vi "相机关闭.vi"(8 "error in (no error)":errorcluster caption="错误输入（无错误）", 11 "数组":T1[](array[typedef])) -> (0 "error out":errorcluster caption="错误输出")   [LabVIEW 2017]
uses:
  <vilib>/userdefined/High Color/IMAQdx.ctl
  <vilib>/vision/driver/NI_Vision_Acquisition_Software.lvlib
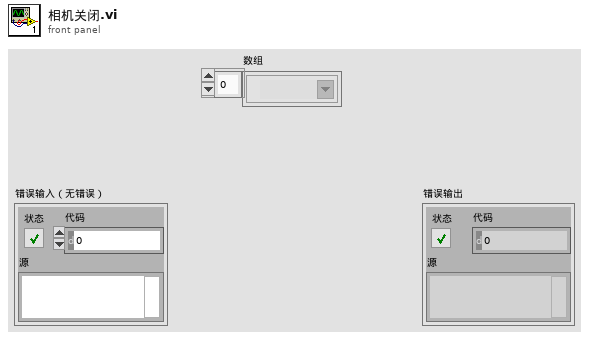
[diagram p1: front panel]
types:
  T1 = typedef "IMAQdx.ctl" = refnum<k21>
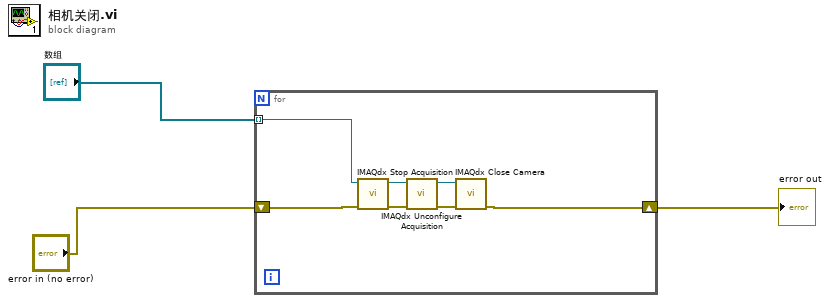
[diagram p0: block diagram]
diagram:
  n1 = for {
    shift-right: [w5] -> w2
    shift-left: "error in (no error)" -> [w6]
    tunnel: "数组" -> [w4] mode=indexing
    n2 = call <vilib>:"IMAQdx Stop Acquisition.vi"("error in"=w6, "Session In"=w4) -> ("error out"=w7:errorcluster, "Session Out"=w8:T1)  [unwired: 8 out]
    n3 = call <vilib>:"IMAQdx Unconfigure Acquisition.vi"("error in"=w7, "Session In"=w8) -> ("error out"=w10:errorcluster, "Session Out"=w9:T1)  [unwired: 8 out]
    n4 = call <vilib>:"IMAQdx Close Camera.vi"("error in"=w10, "Session In"=w9) -> ("error out"=w5:errorcluster)  [unwired: 9 out]
  }
  "error out" <- w2
